vi "API get Sensor AD.vi"(5 "SensorADValueIN":dbl) -> (0 "rtv":bool, 1 "SensorADValueOut":dbl)   [LabVIEW 2011, in "API DYM.lvlib"]
uses:
  API DYM.lvlib
  DyMechnicalPlatform.dll
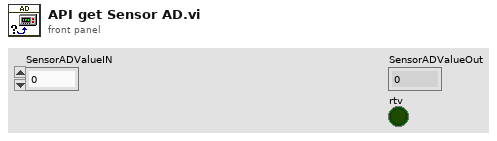
[diagram p1: front panel]
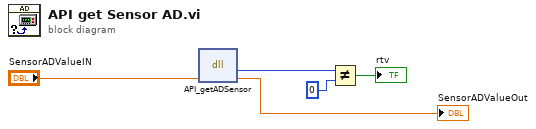
[diagram p0: block diagram]
diagram:
  n1 = dll-call lib="PTH1Xabs D可重构机电平台项目DemoLabViewDYSYSAPIDyMechnicalPlatform.dll" fn="API_getADSensor"("SensorADValue"="SensorADValueIN") -> ("rtv"=w3:i32, "SensorADValue"=→"SensorADValueOut":dbl)  [unwired: 3 in, 2 out]
  n2 = Not Equal?(x=w3, y=0) -> (x != y?=→"rtv":bool)
